vi "LVFunction_Imop_Compute_GaussianParametersComplete.vi"(0 "HasoField in":refnum<class "HasoField.lvclass">, 5 "Path":path, 7 "ArrayOfPSF":refnum<class "SurfaceFloat.lvclass">[](array[class]), 11 "error in (no error)":errorcluster, 12 "degree":sgl, 13 "spottype":enum16{"square", "circle"}(ring)) -> (1 "Gaussian Param":T2, 2 "tab_max_energy":sgl[](array[numeric]), 3 "Data_ mm":T1, 4 "HasoField out":refnum<class "HasoField.lvclass">, 8 "ArrayOfPSF out":refnum<class "SurfaceFloat.lvclass">[](array[class]), 14 "threshold":bool, 15 "error out":errorcluster)   [LabVIEW 2020]
doc: "Complete gaussian parameters function.\n\n--------------------------------------------------------------------------------\n\n<B>config_file_pathIn</B> : Absolute path to the Haso configuration file.\n\n<B>config_file_pathOut</B> : Absolute path to the Haso configuration file.\n\n<B>HasoField</B> : HasoField object.\n\n<B>nb_planes</B> : Number of planes.\n\n<B>waist_position_millimeter</B> : Waist position (mm).\n\n<B>waist_radius_millimeter</B> : Waist radius (mm).\n\n<B>rayleigh_length_millimeter</B> : Rayleigh length (mm).\n\n<B>divergence</B> : Mivergence of the beam.\n\n<B>msquared</B> : m squared parameter.\n\n<B>spot_type</B> : \"square\" or \"circle\" spot shape.\n\n<B>degree</B> : Angle of the square spot shape forms with an horizontal axis (degree).///<\n\n<B>tab_z_cote_mm</B> : Array of z cote (mm) of the different planes.\n\n<B>tab_spot_size_mm</B> : Array of spot size (mm) of the different planes.\n\n<B>tab_psf</B> : Array of computed psf.\n\n<B>threshold</B> : Check whether the entire beam of last processing could be got.\n\n<B>tab_max_energy</B> : Array of max energy of the different planes.\n\n<B>ErrorIn</B> : Error\n\n<B>ErrorOut</B> : Error"
uses:
  HasoField.lvclass
  SurfaceFloat.lvclass
  LVClasse_SurfaceFloat Read SurfaceFloat.vi
  LVClass_HasoField Read HasoField.vi
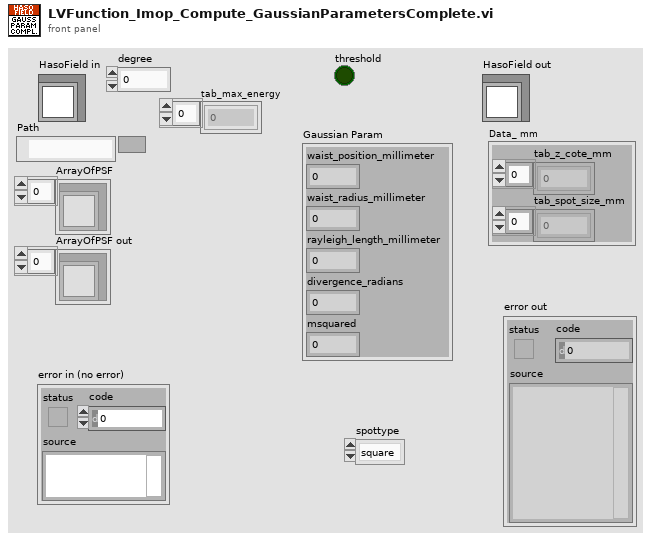
[diagram p1: front panel]
types:
  T1 = cluster{"tab_z_cote_mm":dbl[], "tab_spot_size_mm":dbl[]}
  T2 = cluster{"waist_position_millimeter":sgl, "waist_radius_millimeter":sgl, "rayleigh_length_millimeter":sgl, "divergence_radians":sgl, "msquared":sgl}
  T3 = cluster{"tab_z_cote_mm":sgl[], "tab_spot_size_mm":sgl[]}
  T4 = cluster{"waist_position_millimeter":sgl, "waist_radius_millimeter":sgl, "rayleigh_length_millimeter":sgl, "divergence":sgl, "msquared":sgl}
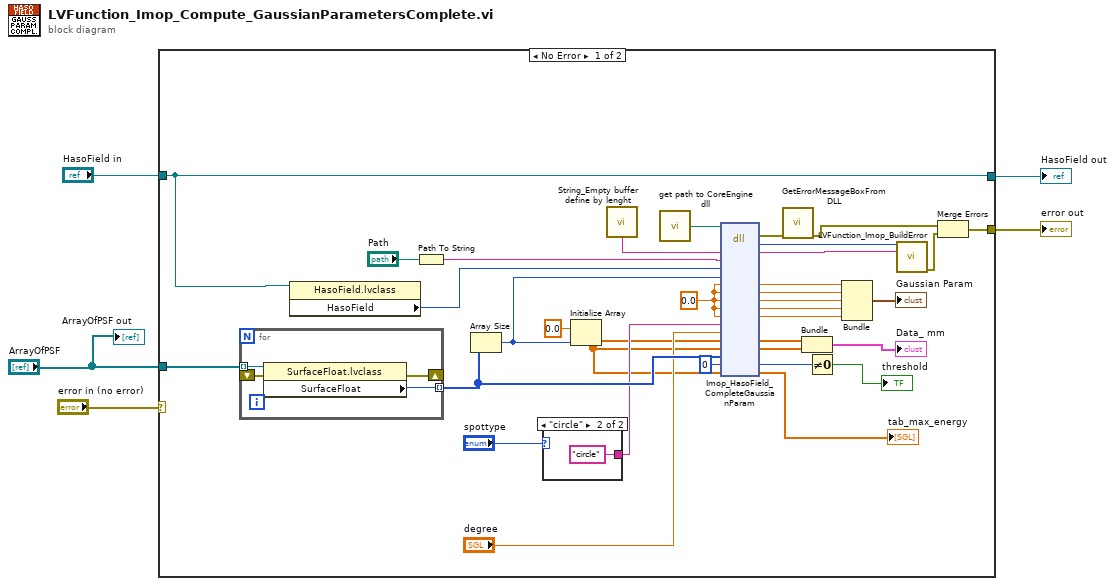
[diagram p0: block diagram]
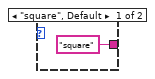
[diagram p2: hidden frame]
diagram:
  n1 = case shown="No Error" "error in (no error)" {
    selector: "error in (no error)" -> [_ w46]
    tunnel: "HasoField in" -> [w22 w47]
    tunnel: [w22 w47] -> w5
    tunnel: [w35 w46] -> w3
    tunnel: "ArrayOfPSF" -> [w16 _]
    frame No Error {
      w29 = sgl 0.0 ("waist_position_millimeter")
      n2 = for {
        tunnel: w16 -> [w44] mode=indexing
        tunnel: [w45] -> w15 mode=indexing
        shift-right: [w42] -> _
        shift-left: _ -> [w43]
        n3 = property class="SurfaceFloat.lvclass"(reference=w44, error in=w43) -> (error out=w42:errorcluster, "SurfaceFloat"=w45:i32)  [unwired: 1 out]
      }
      n4 = property class="HasoField.lvclass"(reference=w22) -> ("HasoField"=w21:i32)  [unwired: 1 in, 2 out]
      n5 = Path To String(path="Path") -> (string=w30:string)
      n6 = Array Size(array=w15) -> (size(s)=w14:i32)
      n7 = case shown="\"circle\"" "spottype" {
        tunnel: ["square" "circle"] -> w11
        frame "square", Default {
        }
        frame "circle" {
        }
      }
      n8 = Initialize Array(0.0 ("element"), w14) -> (w7:dbl[])
      n9 = call "String_Empty buffer define by lenght.vi"() -> ("Empty buffer"=w34:string)  [unwired: 1 in]
      n10 = call "get path to CoreEngine dll.vi"() -> ("path to c_interface_vc100.dll"=w33:path)  [unwired: 12 in, 3 out]
      n11 = dll-call lib="D:/2_trunk/Soft_haso/ImOpCoreEngine4_LV2011/DLLs/ImopEngine4_vc100.dll" fn="Imop_HasoField_CompleteGaussianParam"(path in=w33, "message"=w34, "config file"=w30, "HasoField"=w21, "nb_planes"=w14, "waist_position_millimeter"=w29, "waist_radius_millimeter"=w29, "rayleigh_length_millimeter"=w29, "divergence"=w29, "msquared"=w29, "spottype"=w11, "degree"="degree", "tab_z_cote_mm"=w7, "tab_spot_size_mm"=w7, "tab_psf"=w15, "threshold"=u8 0, "tab_max_energy"=w7) -> (error out=w32:errorcluster, "return type"=w38:i32, "message"=w39:string, "waist_position_millimeter"=w28:sgl, "waist_radius_millimeter"=w27:sgl, "rayleigh_length_millimeter"=w26:sgl, "divergence"=w25:sgl, "msquared"=w24:sgl, "tab_z_cote_mm"=w20:sgl[], "tab_spot_size_mm"=w19:sgl[], "threshold"=w9:u8, "tab_max_energy"=→"tab_max_energy":sgl[])  [unwired: 8 in, 1 out]
      n12 = call "GetErrorMessageBoxFromDLL.vi"("error IN"=w32) -> ("error OUT"=w37:errorcluster)  [unwired: 10 in]
      n13 = Bundle("tab_z_cote_mm"=w20, "tab_spot_size_mm"=w19) -> (→"Data_ mm":T3)  [unwired: 1 in]
      n14 = Not Equal To 0?(x=w9) -> (x != 0?=→"threshold":bool)
      n15 = Bundle("waist_position_millimeter"=w28, "waist_radius_millimeter"=w27, "rayleigh_length_millimeter"=w26, "divergence"=w25, "msquared"=w24) -> (→"Gaussian Param":T4)  [unwired: 1 in]
      n16 = call "LVFunction_Imop_BuildError.vi"("code"=w38, "String to Prepend to source (\"\")"=w39) -> ("error out"=w36:errorcluster)  [unwired: 13 in]
      n17 = Merge Errors(w37, w36) -> (w35:errorcluster)
    }
    frame Error {
    }
  }
  "error out" <- w3
  "HasoField out" <- w5
  "ArrayOfPSF out" <- "ArrayOfPSF"
